vi "Log Data Core.vi"(8 "Error In":errorcluster, 10 "Log Message":T1={"Log Action"=enum."Handle Old Files", "Variant"=variant, "Data Type"=enum."String", "Group Name"="", "Channels Names"=[]}, 11 "TDMS Log In":refnum<class "TDMS Logger.lvclass">) -> (0 "Error Out":errorcluster, 3 "TDMS Log Out":refnum<class "TDMS Logger.lvclass">)   [LabVIEW 2019, in "TDMS Logger.lvlib" / "TDMS Logger.lvclass"]
uses:
  TDMS Logger.lvclass
  _Typedefs/Log Message.ctl
  _Typedefs/Log Action.ctl
  _Typedefs/Data Type.ctl
  TDMS Logger.lvclass/TDMS Logger.ctl
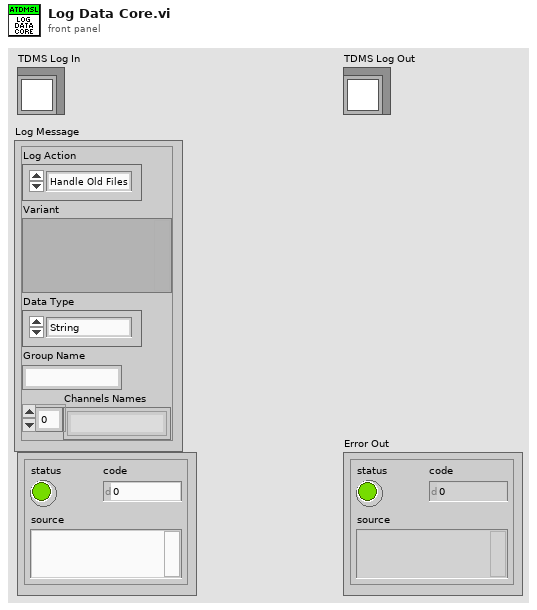
[diagram p1: front panel]
types:
  T1 = typedef "TDMS Logger.lvlib/TDMS Logger.lvclass/Log Message.ctl" = cluster{"Log Action":T2, "Variant":variant, "Data Type":T3, "Group Name":string, "Channels Names":string[]}
  T2 = typedef "TDMS Logger.lvlib/TDMS Logger.lvclass/Log Action.ctl" = enum16{"Handle Old Files", "Status Update", "Stop", "Log Data", "Initialize"}
  T3 = typedef "TDMS Logger.lvlib/TDMS Logger.lvclass/Data Type.ctl" = enum16{"I16", "I8", "String", "U16", "U8", "Waveform", "Double", "Single"}
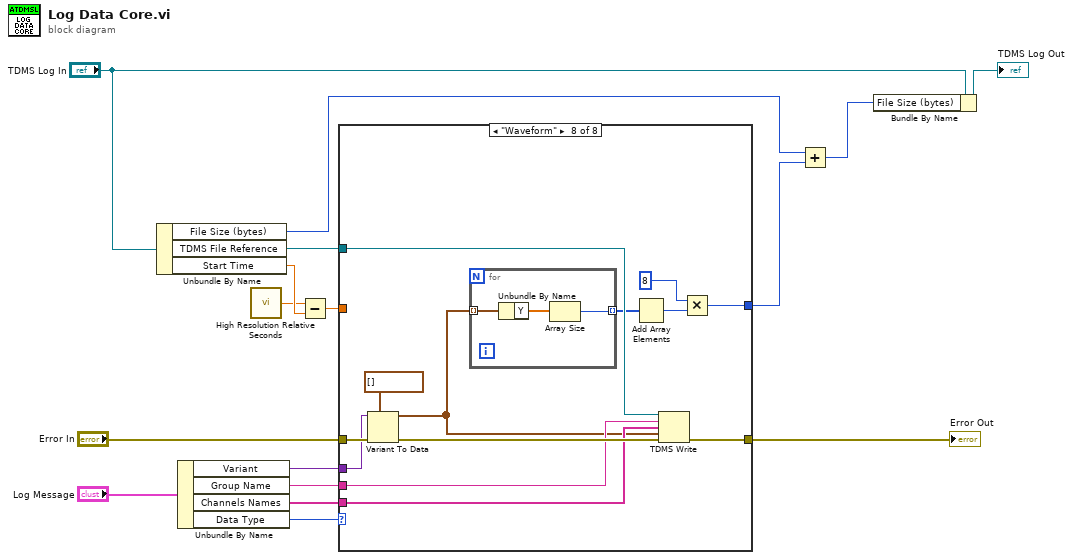
[diagram p0: block diagram]
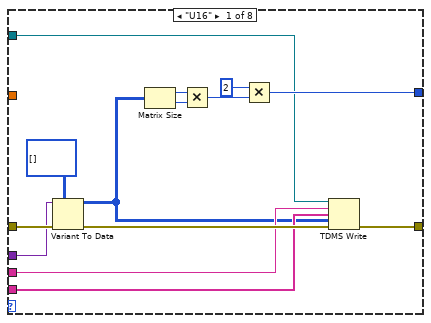
[diagram p2: hidden frame]
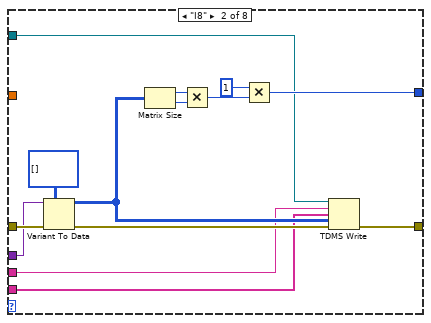
[diagram p3: hidden frame]
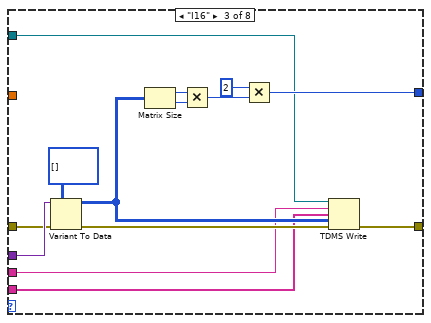
[diagram p4: hidden frame]
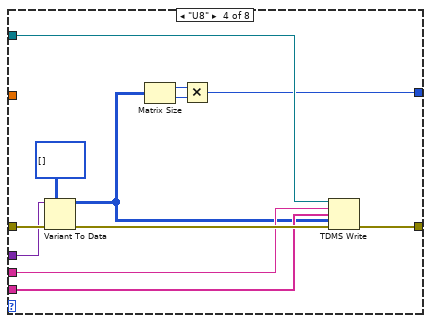
[diagram p5: hidden frame]
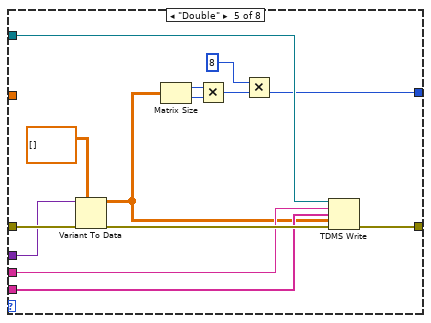
[diagram p6: hidden frame]
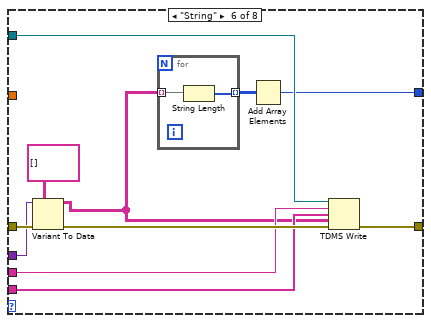
[diagram p7: hidden frame]
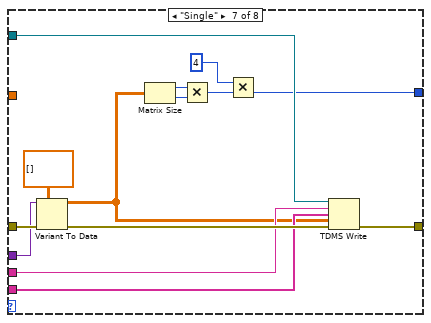
[diagram p8: hidden frame]
diagram:
  n1 = Unbundle By Name("TDMS Log In") -> ("File Size (bytes)"=w5:u64, "TDMS File Reference"=w7:refnum<k34>, "Start Time"=w3:dbl)
  n2 = Unbundle By Name("Log Message") -> ("Variant"=w4:variant, "Group Name"=w9:string, "Channels Names"=w8:string[], "Data Type"=w12:T3)
  n3 = call <vilib>:"High Resolution Relative Seconds.vi"() -> ("relative seconds"=w2:dbl)
  n4 = Subtract(x=w2, y=w3) -> (x-y=w1:dbl)
  n5 = case shown="\"Waveform\"" w12 {
    tunnel: "Error In" -> [w23 w37 w49 w65 w77 w91 w104 w118]
    tunnel: [w26 w44 w58 w66 w79 w92 w106 w122] -> w10
    tunnel: w9 -> [w18 w32 w46 w61 w73 w87 w100 w114]
    tunnel: w8 -> [w19 w31 w45 w60 w72 w86 w99 w113]
    tunnel: w7 -> [w25 w43 w57 w68 w82 w95 w109 w124]
    tunnel: [w24 w42 w56 w67 w81 w94 w108 w123] -> w6
    tunnel: w4 -> [w21 w34 w50 w62 w76 w88 w103 w115]
    tunnel: w1 -> [_ _ _ _ _ _ _ _]
    frame "U16" {
      n6 = Variant To Data(error in=w23, type=u16[][] [] ("element"), Variant=w21) -> (data=w17:u16[][], error out=w22:errorcluster)
      n7 = Matrix Size(0:w17) -> (1:w28:i32, 2:w29:i32)
      n8 = Multiply(x=w28, y=w29) -> (x*y=w27:i32)
      n9 = Multiply(x=2, y=w27) -> (x*y=w26:i32)
      n10 = TDMS Write(0:w25, 5:w18, 7:w19, 9:w17, 11:w22) -> (15:w24:errorcluster)  [unwired: 1 in, 3 out]
    }
    frame "I8" {
      n11 = Variant To Data(error in=w37, type=i8[][] [] ("element"), Variant=w34) -> (data=w33:i8[][], error out=w36:errorcluster)
      n12 = Matrix Size(0:w33) -> (1:w39:i32, 2:w40:i32)
      n13 = Multiply(x=w39, y=w40) -> (x*y=w38:i32)
      n14 = Multiply(x=1, y=w38) -> (x*y=w44:i32)
      n15 = TDMS Write(0:w43, 5:w32, 7:w31, 9:w33, 11:w36) -> (15:w42:errorcluster)  [unwired: 1 in, 3 out]
    }
    frame "I16" {
      n16 = Variant To Data(error in=w49, type=i16[][] [] ("element"), Variant=w50) -> (data=w47:i16[][], error out=w48:errorcluster)
      n17 = Matrix Size(0:w47) -> (1:w53:i32, 2:w54:i32)
      n18 = Multiply(x=w53, y=w54) -> (x*y=w52:i32)
      n19 = Multiply(x=2, y=w52) -> (x*y=w58:i32)
      n20 = TDMS Write(0:w57, 5:w46, 7:w45, 9:w47, 11:w48) -> (15:w56:errorcluster)  [unwired: 1 in, 3 out]
    }
    frame "U8" {
      n21 = Variant To Data(error in=w65, type=u8[][] [] ("element"), Variant=w62) -> (data=w59:u8[][], error out=w64:errorcluster)
      n22 = Matrix Size(0:w59) -> (1:w69:i32, 2:w70:i32)
      n23 = Multiply(x=w69, y=w70) -> (x*y=w66:i32)
      n24 = TDMS Write(0:w68, 5:w61, 7:w60, 9:w59, 11:w64) -> (15:w67:errorcluster)  [unwired: 1 in, 3 out]
    }
    frame "Double" {
      n25 = Variant To Data(error in=w77, type=dbl[][] [], Variant=w76) -> (data=w71:dbl[][], error out=w75:errorcluster)
      n26 = Matrix Size(0:w71) -> (1:w83:i32, 2:w84:i32)
      n27 = Multiply(x=w83, y=w84) -> (x*y=w80:i32)
      n28 = Multiply(x=8, y=w80) -> (x*y=w79:i32)
      n29 = TDMS Write(0:w82, 5:w73, 7:w72, 9:w71, 11:w75) -> (15:w81:errorcluster)  [unwired: 1 in, 3 out]
    }
    frame "String" {
      n30 = Variant To Data(error in=w91, type=string[][] [] ("element"), Variant=w88) -> (data=w85:string[][], error out=w90:errorcluster)
      n31 = for {
        tunnel: w85 -> [w97] mode=indexing
        tunnel: [w96] -> w93 mode=indexing
        n32 = String Length(string=w97) -> (length=w96:i32[])
      }
      n33 = Add Array Elements(numeric array=w93) -> (sum=w92:i32)
      n34 = TDMS Write(0:w95, 5:w87, 7:w86, 9:w85, 11:w90) -> (15:w94:errorcluster)  [unwired: 1 in, 3 out]
    }
    frame "Single" {
      n35 = Variant To Data(error in=w104, type=sgl[][] [] ("element"), Variant=w103) -> (data=w98:sgl[][], error out=w101:errorcluster)
      n36 = Matrix Size(0:w98) -> (1:w110:i32, 2:w111:i32)
      n37 = Multiply(x=w110, y=w111) -> (x*y=w107:i32)
      n38 = Multiply(x=4, y=w107) -> (x*y=w106:i32)
      n39 = TDMS Write(0:w109, 5:w100, 7:w99, 9:w98, 11:w101) -> (15:w108:errorcluster)  [unwired: 1 in, 3 out]
    }
    frame "Waveform" {
      n40 = Variant To Data(error in=w118, type=waveform(dbl)[] [] ("element"), Variant=w115) -> (data=w112:waveform(dbl)[], error out=w117:errorcluster)
      n41 = for {
        tunnel: w112 -> [w127] mode=indexing
        tunnel: [w125] -> w119 mode=indexing
        n42 = Unbundle By Name(w127) -> ("Y"=w126:dbl[])
        n43 = Array Size(array=w126) -> (size(s)=w125:i32)
      }
      n44 = Add Array Elements(numeric array=w119) -> (sum=w120:i32)
      n45 = TDMS Write(0:w124, 5:w114, 7:w113, 9:w112, 11:w117) -> (15:w123:errorcluster)  [unwired: 1 in, 3 out]
      n46 = Multiply(x=8, y=w120) -> (x*y=w122:i32)
    }
  }
  "Error Out" <- w6
  n47 = Add(x=w5, y=w10) -> (x+y=w13:u64)
  n48 = Bundle By Name(cluster="TDMS Log In", "File Size (bytes)"=w13) -> (→"TDMS Log Out":refnum<class "TDMS Logger.lvclass">)
